vi "configure_elo.vi"(11 "VISA Refnum in":refnum<visa-resource-name>) -> (0 "error out":errorcluster, 2 "Operation Mode (0:Constant Current)":u16, 3 "VISA Refnum out":refnum<visa-resource-name>)   [LabVIEW 2019]
uses:
  <instrlib>/Kikusui PLZ 4W Series/Kikusui PLZ 4W Series.lvlib
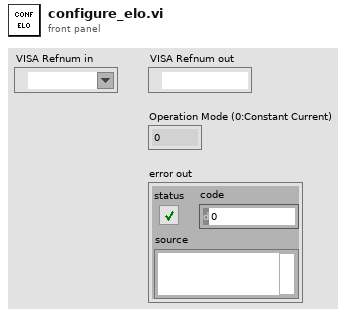
[diagram p1: front panel]
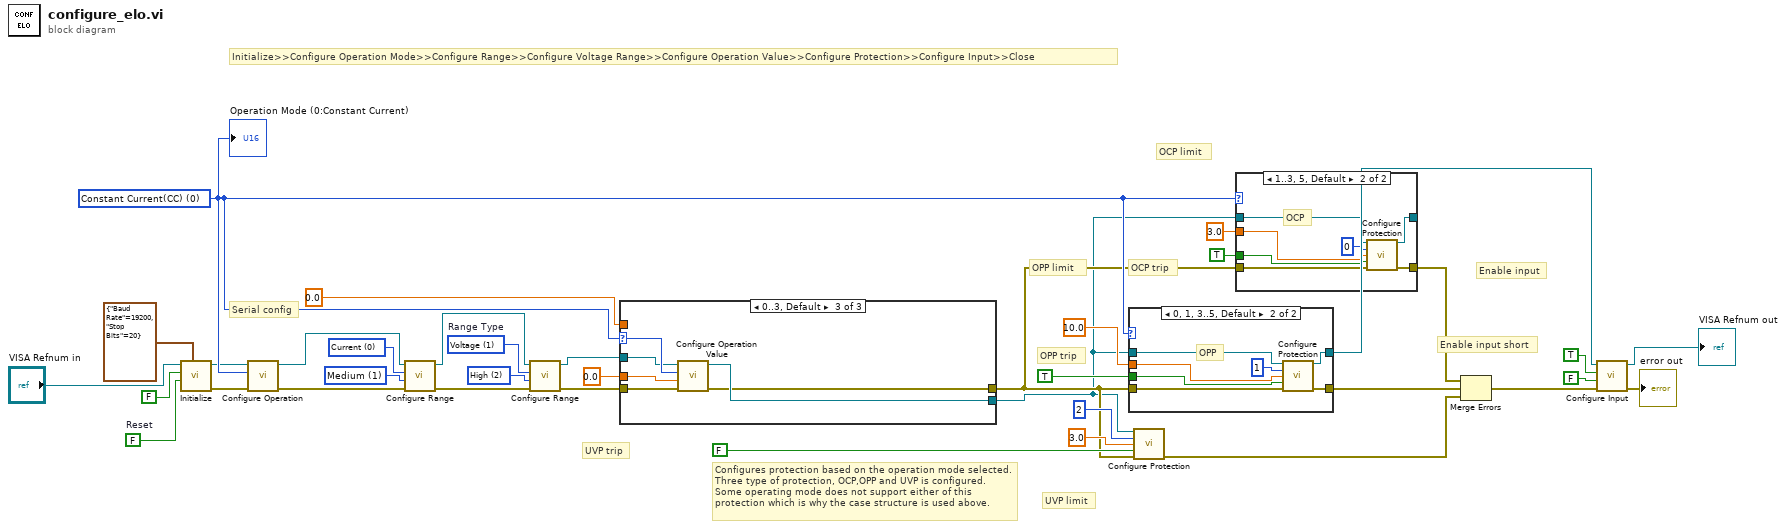
[diagram p0: block diagram]
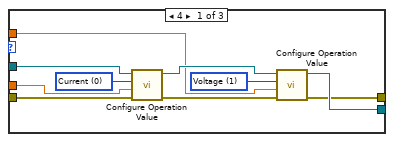
[diagram p4: hidden frame]
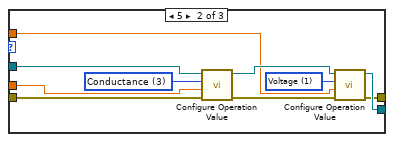
[diagram p5: hidden frame]
diagram:
  w27 = u16 0 items=["Current", "Voltage", "Power", "Conductance"] ("Range Type (0:Current)")
  w13 = u16 2 items=["Low"=0, "High"=2] ("Voltage Range (0:Low)")
  w14 = u16 1 items=["Low", "Medium", "High"] ("Input Range (0:Low)")
  w26 = u16 0 items=["Constant Current(CC)", "Constant Voltage(CV)", "Constant Power(CP)", "Constant Resistance(CR)", "Constant Current & Voltage(CCCV)", "Constant Resistance & Voltage(CRCV)"] ("Operation Mode (0:Constant Current)")
  w22 = FALSE  # Reset
  w12 = u16 1 items=["Current", "Voltage", "Power", "Conductance"]  # Range Type
  # "Serial config"
  # "UVP trip"
  # "UVP limit"
  # "OPP trip"
  # "OPP limit"
  # "OCP trip"
  # "OCP limit"
  # "Enable input short"
  # "Enable input"
  # "Configures protection based on the operation mode selected. Three type of protection, OCP,OPP and UVP is configured. Some operating mode does not support either of this protection which is why the case structure is used above."
  # "Initialize>>Configure Operation Mode>>Configure Range>>Configure Voltage Range>>Configure Operation Value>>Configure Protection>>Configure Input>>Close"
  n1 = call <instrlib>:"Initialize.vi"("Serial Configuration"=cluster{"Baud Rate":u32, "Stop Bits":u16} {"Baud Rate"=19200, "Stop Bits"=20}, "Reset (True)"=w22, "ID Query (True)"=FALSE, "VISA resource name"="VISA Refnum in") -> ("error out"=w5:errorcluster, "VISA resource name out"=w4:refnum<visa-resource-name>)  [unwired: 6 in]
  n2 = call <instrlib>:"Configure Operation.vi"("error in (no error)"=w5, "Operation Mode (0:Constant Current)"=w26, "VISA resource name"=w4) -> ("error out"=w11:errorcluster, "VISA resource name out"=w10:refnum<visa-resource-name>)  [unwired: 7 in]
  n3 = call <instrlib>:"Configure Range.vi"("error in (no error)"=w11, "Range (0:Low)"=w14, "Range Type (0:Current)"=w27, "VISA resource name"=w10) -> ("error out"=w9:errorcluster, "VISA resource name out"=w8:refnum<visa-resource-name>)  [unwired: 6 in]
  n4 = call <instrlib>:"Configure Range.vi"("error in (no error)"=w9, "Range (0:Low)"=w13, "Range Type (0:Current)"=w12, "VISA resource name"=w8) -> ("error out"=w7:errorcluster, "VISA resource name out"=w6:refnum<visa-resource-name>)  [unwired: 6 in]
  n5 = case shown="0..3, Default" w26 {
    selector: w26 -> [_ _ w60]
    tunnel: 0.0 ("Input Value(0)") -> [w42 w50 w63]
    tunnel: w6 -> [w47 w55 w59]
    tunnel: w7 -> [w46 w54 w58]
    tunnel: [w43 w53 w62] -> w15
    tunnel: [w40 w52 w61] -> w16
    tunnel: 0.0 ("Voltage Value (0)") -> [w41 w51 _]
    frame 4 {
      w38 = u16 1 items=["Current", "Voltage", "Power", "Conductance"] ("Value Type (0:Current)")
      w39 = u16 0 items=["Current", "Voltage", "Power", "Conductance"] ("Value Type (0:Current)")
      n6 = call <instrlib>:"Configure Operation Value.vi"("error in (no error)"=w46, "Values (0)"=w42, "Value Type (0:Current)"=w39, "VISA resource name"=w47) -> ("error out"=w44:errorcluster, "VISA resource name out"=w45:refnum<visa-resource-name>)  [unwired: 6 in]
      n7 = call <instrlib>:"Configure Operation Value.vi"("error in (no error)"=w44, "Values (0)"=w41, "Value Type (0:Current)"=w38, "VISA resource name"=w45) -> ("error out"=w40:errorcluster, "VISA resource name out"=w43:refnum<visa-resource-name>)  [unwired: 6 in]
    }
    frame 5 {
      w48 = u16 1 items=["Current", "Voltage", "Power", "Conductance"] ("Value Type (0:Current)")
      w49 = u16 3 items=["Current", "Voltage", "Power", "Conductance"] ("Value Type (0:Current)")
      n8 = call <instrlib>:"Configure Operation Value.vi"("error in (no error)"=w54, "Values (0)"=w50, "Value Type (0:Current)"=w49, "VISA resource name"=w55) -> ("error out"=w56:errorcluster, "VISA resource name out"=w57:refnum<visa-resource-name>)  [unwired: 6 in]
      n9 = call <instrlib>:"Configure Operation Value.vi"("error in (no error)"=w56, "Values (0)"=w51, "Value Type (0:Current)"=w48, "VISA resource name"=w57) -> ("error out"=w52:errorcluster, "VISA resource name out"=w53:refnum<visa-resource-name>)  [unwired: 6 in]
    }
    frame 0..3, Default {
      n10 = call <instrlib>:"Configure Operation Value.vi"("error in (no error)"=w58, "Values (0)"=w63, "Value Type (0:Current)"=w60, "VISA resource name"=w59) -> ("error out"=w61:errorcluster, "VISA resource name out"=w62:refnum<visa-resource-name>)  [unwired: 6 in]
    }
  }
  n11 = case shown="0, 1, 3..5, Default" w26 {
    tunnel: w15 -> [w65 w72]
    tunnel: w16 -> [w64 w71]
    tunnel: [w65 w70] -> w20
    tunnel: [w64 w69] -> w21
    tunnel: 10.0 ("OPP Limit (0)") -> [_ w68]
    tunnel: TRUE ("OPP Trip (Disable)") -> [_ w66]
    frame 2 {
    }
    frame 0, 1, 3..5, Default {
      # "OPP"
      n12 = call <instrlib>:"Configure Protection.vi"("VISA resource name"=w72, "Protection Type (0:OCP)"=1, "Protection Limit (0)"=w68, "Enable Trip (Disable)"=w66, "error in (no error)"=w71) -> ("VISA resource name out"=w70:refnum<visa-resource-name>, "error out"=w69:errorcluster)  [unwired: 9 in]
    }
  }
  n13 = call <instrlib>:"Configure Protection.vi"("VISA resource name"=w15, "Protection Type (0:OCP)"=2, "Protection Limit (0)"=3.0 ("UVP Limit (0)"), "Enable Trip (Disable)"=FALSE ("UVP (Enable)"), "error in (no error)"=w16) -> ("error out"=w18:errorcluster)  [unwired: 9 in, 1 out]
  n14 = case shown="1..3, 5, Default" w26 {
    tunnel: w15 -> [w74 w81]
    tunnel: w16 -> [w73 w80]
    tunnel: [w74 w79] -> _
    tunnel: [w73 w78] -> w17
    tunnel: 3.0 ("OCP Limit (0)") -> [_ w77]
    tunnel: TRUE ("OCP Trip (Disable)") -> [_ w75]
    frame 0, 4 {
    }
    frame 1..3, 5, Default {
      # "OCP"
      n15 = call <instrlib>:"Configure Protection.vi"("VISA resource name"=w81, "Protection Type (0:OCP)"=0, "Protection Limit (0)"=w77, "Enable Trip (Disable)"=w75, "error in (no error)"=w80) -> ("VISA resource name out"=w79:refnum<visa-resource-name>, "error out"=w78:errorcluster)  [unwired: 9 in]
    }
  }
  n16 = Merge Errors(w17, w21, w18) -> (w19:errorcluster)
  n17 = call <instrlib>:"Configure Input.vi"("error in (no error)"=w19, "Enable Input Short (Disable)"=FALSE, "Enable Input (Enable)"=TRUE, "VISA resource name"=w20) -> ("error out"=→"error out":errorcluster, "VISA resource name out"=→"VISA Refnum out":refnum<visa-resource-name>)  [unwired: 6 in]
  "Operation Mode (0:Constant Current)" <- w26
